vi "CmdExe.Launch Executable with Timeout, Abort, and Error Checks_V3.vi"(4 "StdIn":string, 5 "Cmd IN Ref":refnum<vi>, 6 "Setup":T1={"Timeout (s)"=60.0, "Show Cmd Win"=FALSE, "Error Check"={"StdOut_Ck"=FALSE, "StdOutErrMsgs"=["Error", "Unable to find device "], "StdErr_Ck"=FALSE, "RtnCode_Ck"=FALSE, "RtnCodePASS"=0}, "Log_En"=FALSE, "LogFileName"="", "LogDir"=path ""}, 7 "Output Ref":refnum<vi>, 8 "error in (no error)":errorcluster, 9 "Ignore StdErr":bool, 10 "Args":string, 11 "Executable":path=path "C:/MTE/FW Load and Display Cal/Config/Bin/utahev_0_7/lighthouse_configtool.exe") -> (0 "error out":errorcluster, 1 "Duration(s)":dbl, 2 "return code":i32, 3 "Data Out":string)   [LabVIEW 2024]
uses:
  CmdExe.Setup Params.ctl
  CmdExe.Output Error Check Setup.ctl
  Errors/Error.Error Code List.ctl
  Errors.lvlib
  <vilib>/KATE/Time/Time Utils.lvlib
  <vilib>/KATE/Files/File Utils.lvlib
panel:
  out "Cmd":string
  out "Done":bool
  # "Launch Exe"
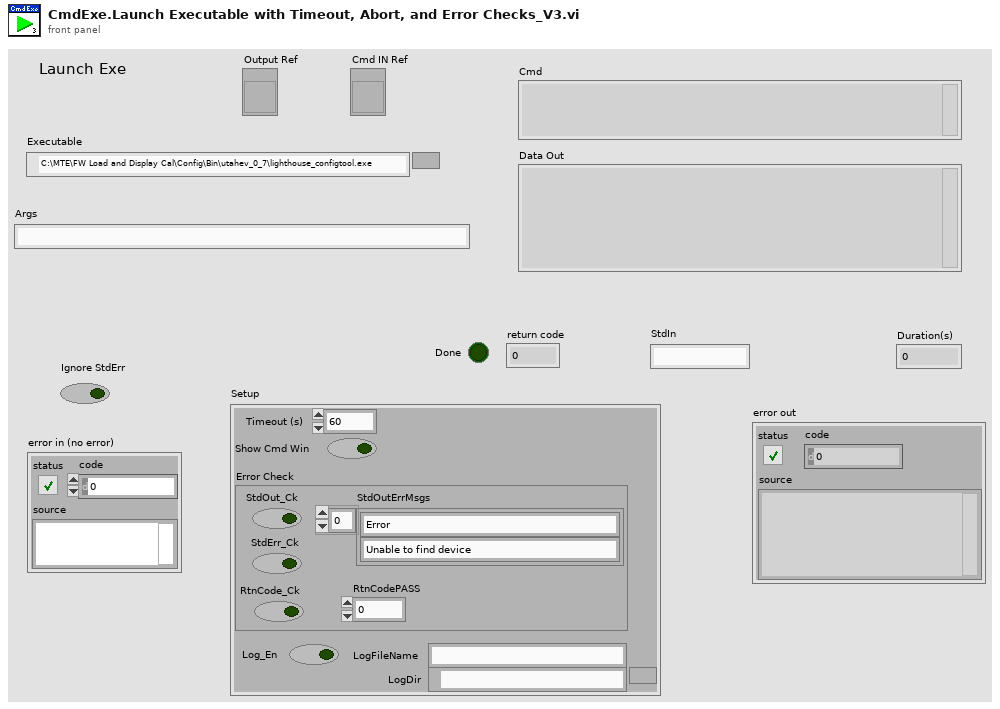
[diagram p1: front panel]
types:
  T1 = typedef "CmdExe.Setup Params.ctl" = cluster{"Timeout (s)":dbl, "Show Cmd Win":bool, "Error Check":T2, "Log_En":bool, "LogFileName":string, "LogDir":path}
  T2 = typedef "CmdExe.Output Error Check Setup.ctl" = cluster{"StdOut_Ck":bool, "StdOutErrMsgs":string[], "StdErr_Ck":bool, "RtnCode_Ck":bool, "RtnCodePASS":i32}
  T3 = enum16{"open", "replace", "create", "open or create", "replace or create", "replace or create with confirmation"}
  T4 = cluster{"Exe":string, "StdOut":string, "StdError":string, "LogFile":path, "Args":string, "TimedOut":bool, "RtnCode":i32, "LogEn":bool}
  T5 = typedef "EQMF.lvlib/Errors.lvlib/Error.Error Code List.ctl" = i32
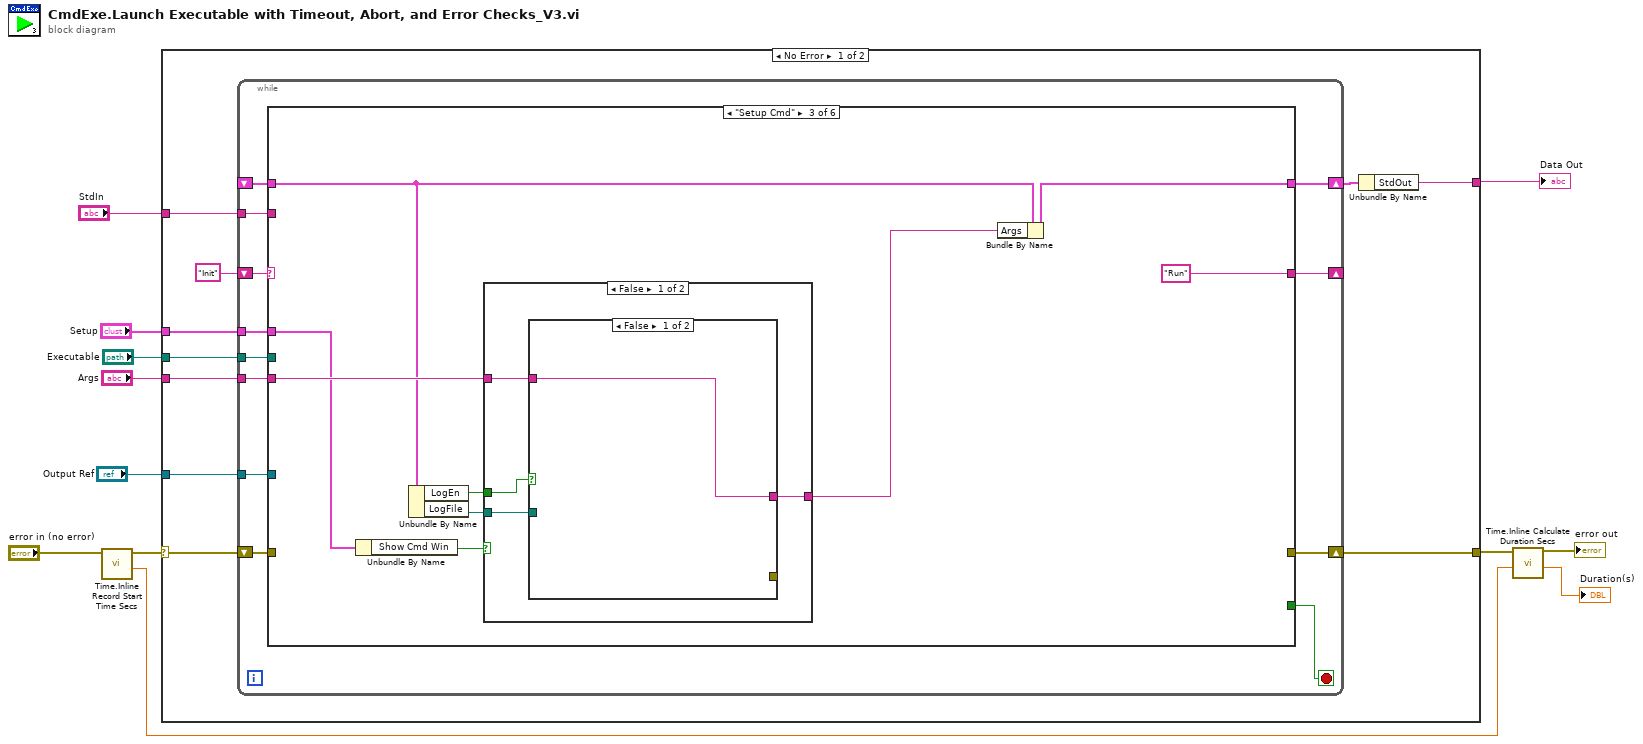
[diagram p0: block diagram]
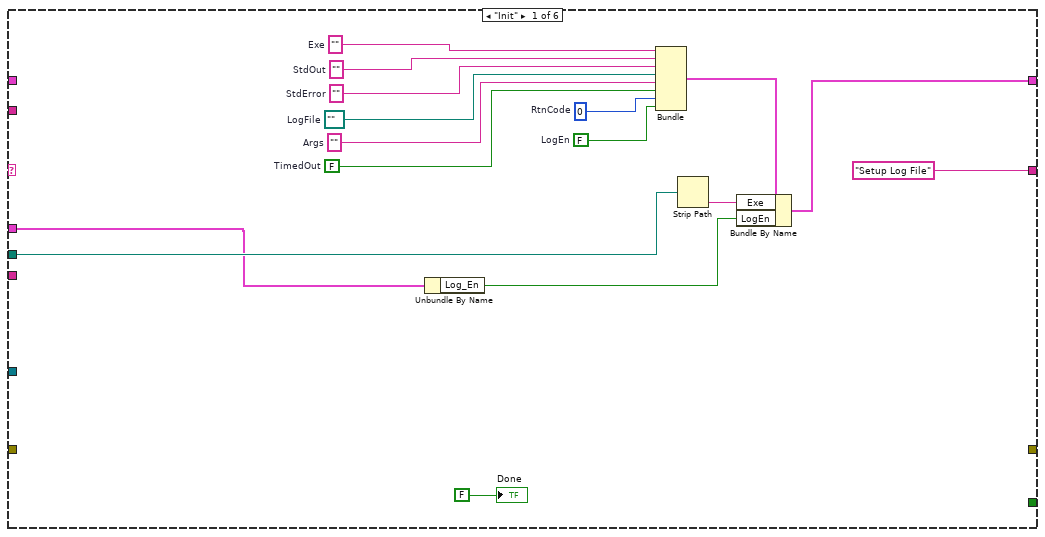
[diagram p2: hidden frame]
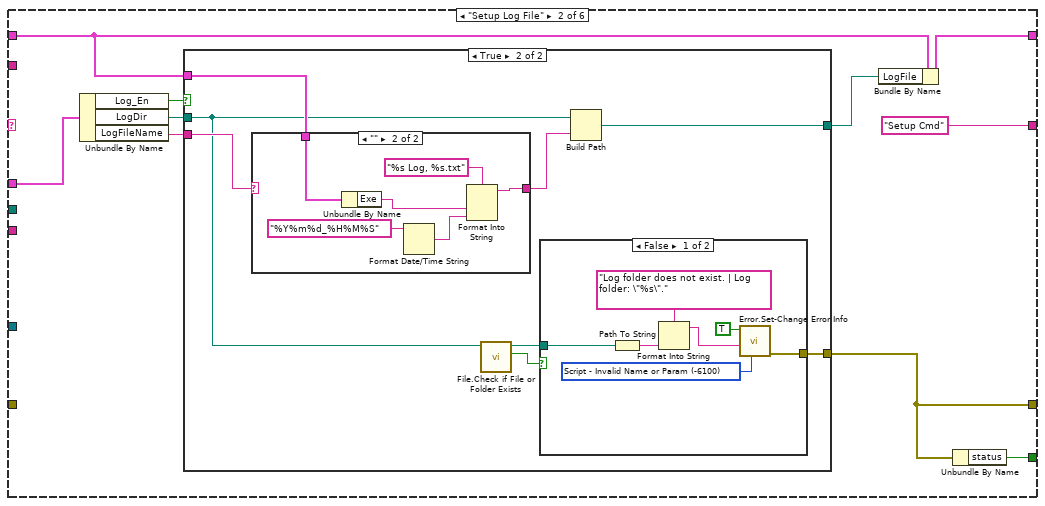
[diagram p3: hidden frame]
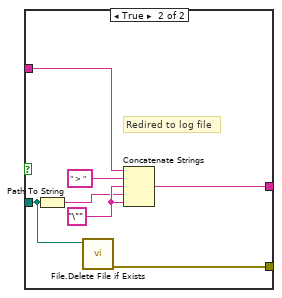
[diagram p7: hidden frame]
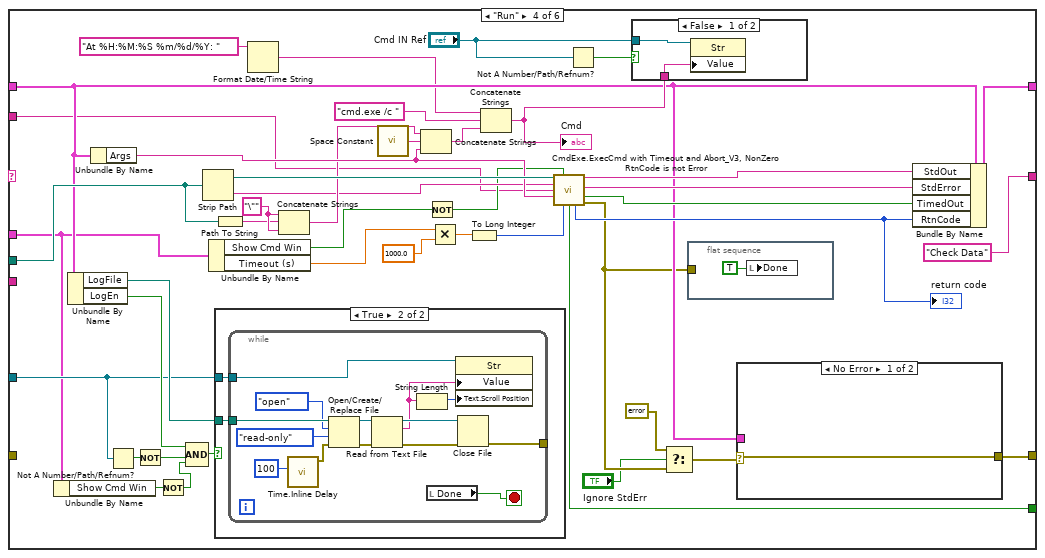
[diagram p9: hidden frame]
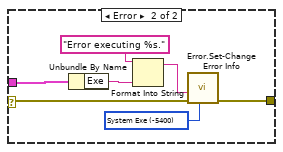
[diagram p10: hidden frame]
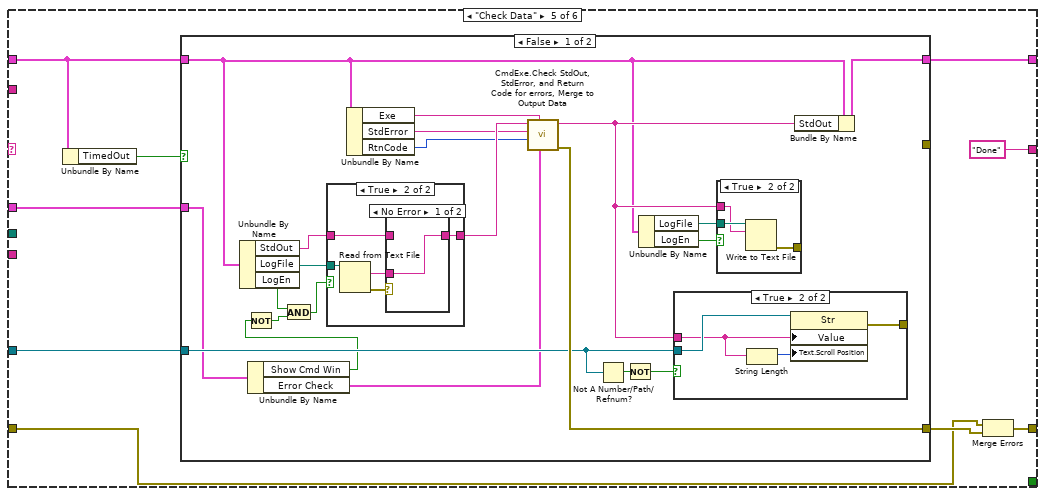
[diagram p13: hidden frame]
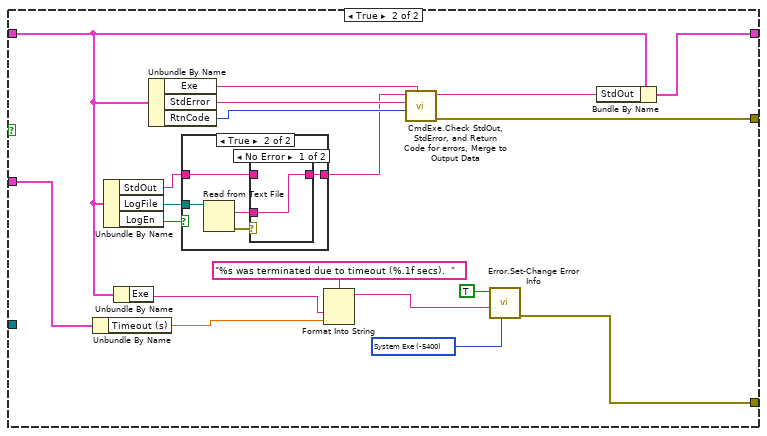
[diagram p18: hidden frame]
diagram:
  n1 = call <vilib>:"Time.Inline Record Start Time Secs.vi"("Error In Upper"="error in (no error)") -> ("Start(s)"=w9:dbl, "Error Out Upper"=w12:errorcluster)  [unwired: 8 in, 1 out]
  n2 = case shown="No Error" w12 {
    selector: w12 -> [w21 w252]
    tunnel: [w20 w252] -> w11
    tunnel: [w18 _] -> w10
    tunnel: "Executable" -> [w17 _]
    tunnel: "Args" -> [w16 _]
    tunnel: "Setup" -> [w15 _]
    tunnel: "Output Ref" -> [w14 _]
    tunnel: "StdIn" -> [w13 _]
    frame No Error {
      n3 = while {
        shift-right: [w32] -> w19
        shift-left: _ -> [w31]
        shift-right: [w24] -> _
        shift-left: "Init" -> [w34]
        shift-right: [w30] -> w20
        shift-left: w21 -> [w33]
        tunnel: w17 -> [w28]
        tunnel: w16 -> [w27]
        tunnel: w15 -> [w26]
        tunnel: w14 -> [w25]
        tunnel: w13 -> [w23]
        stop <- w29 stop-if-true
        n4 = case shown="\"Setup Cmd\"" w34 {
          tunnel: ["Setup Log File" "Setup Cmd" "Run" "Check Data" "Done" "Done"] -> w24
          tunnel: w33 -> [_ _ _ _ w176 w248]
          tunnel: [w39 w59 w90 w148 w184 w249] -> w32
          tunnel: [_ w52 _ w116 w178 w248] -> w30
          tunnel: w31 -> [_ w57 w85 w115 w182 w249]
          tunnel: [_ w51 _ w144 _ TRUE] -> w29
          tunnel: w28 -> [w42 _ _ w129 _ _]
          tunnel: w27 -> [_ _ w88 _ _ _]
          tunnel: w26 -> [w36 w56 w84 w110 w180 _]
          tunnel: w25 -> [_ _ _ w117 w183 _]
          tunnel: w23 -> [_ _ _ w107 _ _]
          frame "Init" {
            w37 = FALSE  # LogEn
            w38 = 0  # RtnCode
            w43 = FALSE  # TimedOut
            w44 = ""  # Args
            w45 = path ""  # LogFile
            w46 = ""  # StdError
            w47 = ""  # StdOut
            w49 = ""  # Exe
            n5 = Unbundle By Name(w36) -> ("Log_En"=w35:bool)
            n6 = Bundle("Exe"=w49, "StdOut"=w47, "StdError"=w46, "LogFile"=w45, "Args"=w44, "TimedOut"=w43, "RtnCode"=w38, "LogEn"=w37) -> (w40:T4)  [unwired: 1 in]
            n7 = Strip Path(path=w42) -> (name=w41:string)  [unwired: 1 out]
            n8 = Bundle By Name(cluster=w40, "Exe"=w41, "LogEn"=w35) -> (w39:T4)
            "Done" <- FALSE ("Done")
          }
          frame "Setup Log File" {
            n9 = Unbundle By Name(w56) -> ("Log_En"=w55:bool, "LogDir"=w54:path, "LogFileName"=w53:string)
            n10 = case shown="True" w55 {
              tunnel: [_ w68] -> w58
              tunnel: w57 -> [_ w66]
              tunnel: w54 -> [_ w62]
              tunnel: w53 -> [_ w65]
              tunnel: [_ w61] -> w52
              frame False {
              }
              frame True {
                n11 = case shown="\"\"" w65 {
                  selector: w65 -> [w76 _]
                  tunnel: [w76 w79] -> w67
                  tunnel: w66 -> [_ w78]
                  frame Default {
                  }
                  frame "" {
                    n12 = Unbundle By Name(w78) -> ("Exe"=w77:string)
                    n13 = Format Date/Time String(time format string (%c)="%Y%m%d_%H%M%S") -> (date/time string=w82:string)  [unwired: 2 in]
                    n14 = Format Into String(format string="%s Log, %s.txt", w77, w82) -> (resulting string=w79:string)  [unwired: 2 in, 1 out]
                  }
                }
                n15 = call <vilib>:"File.Check if File or Folder Exists.vi"("Path"=w62) -> ("Exists"=w63:bool, "Dup Path"=w64:path)  [unwired: 6 in, 3 out]
                n16 = case shown="False" w63 {
                  tunnel: [w69 _] -> w61
                  tunnel: w64 -> [w73 _]
                  frame False {
                    w71 = T5 -6100 items=["No Error"=0, "Abort"=-2, "Misc"=-5000, "Fixture Error"=-5100, "File IO - General"=-5200, "FIle IO - Config Error"=-5201, "Instrument - General"=-5300, "Instrument - Serial Com"=-5301, "Instrument - Camera"=-5302, "Instrument - PS"=-5303, "Instrument - Oscilloscope"=-5304, "Instrument - Function Gen"=-5305, "Instrument - Load"=-5306, "Instrument - Meter"=-5307, "Instrument - Power Control"=-5308, "Instrument - Motion"=-5309, "Instrument - RF"=-5310, "System Exe"=-5400, "Image Processing"=-5500, "Communication"=-5600, "Script - Syntax Error"=-6000, "Script - Invalid Name or Param"=-6100, "Script - Timeout"=-6200, "Invalid Data"=-6300] ("Std Code")
                    n17 = Path To String(path=w73) -> (string=w74:string)
                    n18 = Format Into String(format string="Log folder does not exist. | Log folder: \"%s\".", w74) -> (resulting string=w70:string)  [unwired: 2 in, 1 out]
                    n19 = call "Error.Set-Change Error Info.vi"("Std Code"=w71, "Description"=w70, "Set Error"=TRUE) -> ("error out"=w69:errorcluster)  [unwired: 8 in]
                  }
                  frame True {
                    # "Folders exist.\nNo error."
                  }
                }
                n20 = Build Path(base path=w62, name or relative path=w67) -> (appended path=w68:path)
              }
            }
            n21 = Bundle By Name(cluster=w57, "LogFile"=w58) -> (w59:T4)
            n22 = Unbundle By Name(w52) -> ("status"=w51:bool)
          }
          frame "Setup Cmd" {
            n23 = Unbundle By Name(w84) -> ("Show Cmd Win"=w83:bool)
            n24 = Unbundle By Name(w85) -> ("LogEn"=w86:bool, "LogFile"=w89:path)
            n25 = case shown="False" w83 {
              tunnel: w89 -> [w95 _]
              tunnel: w88 -> [w94 w104]
              tunnel: [w93 w104] -> w87
              tunnel: w86 -> [w92 _]
              frame False {
                n26 = case shown="False" w92 {
                  tunnel: w95 -> [_ w98]
                  tunnel: w94 -> [w96 w100]
                  tunnel: [w96 w99] -> w93
                  tunnel: [_ w97] -> _
                  frame False {
                  }
                  frame True {
                    w103 = "\""
                    # "Redired to log file"
                    n27 = Path To String(path=w98) -> (string=w102:string)
                    n28 = call "File.Delete File if Exists.vi"("Path"=w98) -> ("error out"=w97:errorcluster)  [unwired: 9 in, 1 out]
                    n29 = Concatenate Strings(w100, " > ", w103, w102, w103) -> (w99:string)
                  }
                }
              }
              frame True {
              }
            }
            n30 = Bundle By Name(cluster=w85, "Args"=w87) -> (w90:T4)
          }
          frame "Run" {
            w130 = "\""
            n31 = Unbundle By Name(w110) -> ("Show Cmd Win"=w109:bool)
            n32 = Unbundle By Name(w115) -> ("LogFile"=w138:path, "LogEn"=w122:bool)
            n33 = Unbundle By Name(w115) -> ("Args"=w131:string)
            n34 = Not A Number/Path/Refnum?(number/path/refnum=w117) -> (NaN/Path/Refnum?=w125:bool)
            n35 = Not(x=w125) -> (.not. x?=w124:bool)
            n36 = Not(x=w109) -> (.not. x?=w108:bool)
            n37 = Compound Arithmetic op=AND(w122, w124, w108) -> (w123:bool)
            n38 = Strip Path(path=w129) -> (stripped path=w137:path, name=w126:string)
            n39 = Unbundle By Name(w110) -> ("Show Cmd Win"=w120:bool, "Timeout (s)"=w121:dbl)
            n40 = Path To String(path=w129) -> (string=w128:string)
            n41 = case shown="True" w123 {
              tunnel: w138 -> [_ w160]
              tunnel: w117 -> [_ w161]
              frame False {
              }
              frame True {
                n42 = while {
                  tunnel: w161 -> [w167]
                  tunnel: w160 -> [w171]
                  tunnel: [w170] -> _
                  stop <- w166 stop-if-true
                  n43 = call <vilib>:"Time.Inline Delay.vi"("Wait(ms)"=u32 100) -> ("error out top"=w164:errorcluster)  [unwired: 9 in, 1 out]
                  n44 = Open/Create/Replace File(file path (use dialog)=w171, error in=w164, operation (0:open)=T3."open", access (0:read/write)=enum16{"read/write", "read-only", "write-only"}."read-only") -> (refnum out=w172:refnum<file>, error out=w175:errorcluster)  [unwired: 2 in, 1 out]
                  n45 = Read from Text File(file (use dialog)=w172, error in=w175) -> (refnum out=w173:refnum<file>, text=w163:string, error out=w174:errorcluster)  [unwired: 2 in, 1 out]
                  n46 = String Length(string=w163) -> (length=w162:i32)
                  n47 = local read "Done"() -> (w166:bool)
                  n48 = property class="Str"(reference=w167, "Value"=w163, "Text.Scroll Position"=w162) -> ()  [unwired: 1 in, 2 out]
                  n49 = Close File(refnum=w173, error in=w174) -> (error out=w170:errorcluster)  [unwired: 1 out]
                }
              }
            }
            n50 = Format Date/Time String(time format string (%c)="At %H:%M:%S %m/%d/%Y: ") -> (date/time string=w105:string)  [unwired: 2 in]
            n51 = Concatenate Strings(w130, w128, w130) -> (w127:string)
            n52 = call <vilib>:"Space Constant.vi"() -> ("String"=w134:string)
            n53 = Concatenate Strings(w127, w134, w131) -> (w135:string)
            n54 = Not(x=w120) -> (.not. x?=w119:bool)
            n55 = Multiply(x=w121, y=1000.0) -> (x*y=w143:dbl)
            n56 = To Long Integer(number=w143) -> (32bit integer=w141:i32)
            n57 = Concatenate Strings(w105, "cmd.exe /c ", w135) -> (w133:string)
            "Cmd" <- w133
            n58 = call "CmdExe.ExecCmd with Timeout and Abort_V3, NonZero RtnCode is not Error.vi"("Working Dir"=w137, "Run minimized? (T)"=w119, "Executable"=w126, "StdIn"=w107, "Arguements"=w131, "Timeout ms(-1)"=w141) -> ("STD OUT"=w118:string, "STD ERR"=w147:string, "Timed Out"=w146:bool, "Aborted"=w144:bool, "return code"=w132:i32, "error out"=w114:errorcluster)  [unwired: 4 in]
            "return code" <- w132
            n59 = Not A Number/Path/Refnum?(number/path/refnum="Cmd IN Ref") -> (NaN/Path/Refnum?=w140:bool)
            n60 = case shown="False" w140 {
              tunnel: "Cmd IN Ref" -> [w159 _]
              tunnel: w133 -> [w158 _]
              frame False {
                n61 = property class="Str"(reference=w159, "Value"=w158) -> ()  [unwired: 1 in, 2 out]
              }
              frame True {
              }
            }
            n62 = Select(t=errorcluster {"status"=FALSE, "code"=0, "source"=""}, s="Ignore StdErr", f=w114) -> (s? t:f=w113:errorcluster)
            n63 = flat-sequence {
              tunnel: w114 -> [_]
              frame #0 {
                n64 = local write "Done"(TRUE ("Done")) -> ()
              }
            }
            n65 = case shown="No Error" w113 {
              selector: w113 -> [w149 w152]
              tunnel: [w149 w151] -> w116
              tunnel: w115 -> [_ w150]
              frame No Error {
              }
              frame Error {
                w154 = T5 -5400 items=["No Error"=0, "Abort"=-2, "Misc"=-5000, "Fixture Error"=-5100, "File IO - General"=-5200, "FIle IO - Config Error"=-5201, "Instrument - General"=-5300, "Instrument - Serial Com"=-5301, "Instrument - Camera"=-5302, "Instrument - PS"=-5303, "Instrument - Oscilloscope"=-5304, "Instrument - Function Gen"=-5305, "Instrument - Load"=-5306, "Instrument - Meter"=-5307, "Instrument - Power Control"=-5308, "Instrument - Motion"=-5309, "Instrument - RF"=-5310, "System Exe"=-5400, "Image Processing"=-5500, "Communication"=-5600, "Script - Syntax Error"=-6000, "Script - Invalid Name or Param"=-6100, "Script - Timeout"=-6200, "Invalid Data"=-6300] ("Std Code")
                n66 = Unbundle By Name(w150) -> ("Exe"=w155:string)
                n67 = Format Into String(format string="Error executing %s.", w155) -> (resulting string=w153:string)  [unwired: 2 in, 1 out]
                n68 = call "Error.Set-Change Error Info.vi"("Std Code"=w154, "error in"=w152, "Description"=w153) -> ("error out"=w151:errorcluster)  [unwired: 8 in]
              }
            }
            n69 = Bundle By Name(cluster=w115, "StdOut"=w118, "StdError"=w147, "TimedOut"=w146, "RtnCode"=w132) -> (w148:T4)
          }
          frame "Check Data" {
            n70 = Unbundle By Name(w182) -> ("TimedOut"=w181:bool)
            n71 = case shown="False" w181 {
              tunnel: [w205 w227] -> w184
              tunnel: w182 -> [w189 w221]
              tunnel: [w200 w232] -> w177
              tunnel: w183 -> [w197 _]
              tunnel: w180 -> [w194 w237]
              tunnel: [_ w222] -> _
              frame False {
                n72 = Unbundle By Name(w189) -> ("StdOut"=w195:string, "LogFile"=w204:path, "LogEn"=w188:bool)
                n73 = Unbundle By Name(w194) -> ("Show Cmd Win"=w186:bool, "Error Check"=w193:T2)
                n74 = Not(x=w186) -> (.not. x?=w187:bool)
                n75 = And(x=w188, y=w187) -> (x .and. y?=w185:bool)
                n76 = case shown="True" w185 {
                  tunnel: w204 -> [_ w218]
                  tunnel: [w213 w216] -> w203
                  tunnel: w195 -> [w213 w214]
                  frame False {
                    (unwired) TRUE
                  }
                  frame True {
                    n77 = Read from Text File(file (use dialog)=w218) -> (text=w215:string, error out=w217:errorcluster)  [unwired: 3 in, 2 out]
                    n78 = case shown="No Error" w217 {
                      tunnel: [w219 w220] -> w216
                      tunnel: w215 -> [w219 _]
                      tunnel: w214 -> [_ w220]
                      frame No Error {
                      }
                      frame Error {
                      }
                    }
                  }
                }
                n79 = Unbundle By Name(w189) -> ("Exe"=w196:string, "StdError"=w202:string, "RtnCode"=w201:i32)
                n80 = call "CmdExe.Check StdOut, StdError, and Return Code for errors, Merge to Output Data.vi"("Error Check"=w193, "App Name"=w196, "Return Code"=w201, "StdError"=w202, "StdOut"=w203) -> ("error out"=w200:errorcluster, "Output Data"=w190:string)  [unwired: 5 in]
                n81 = Not A Number/Path/Refnum?(number/path/refnum=w197) -> (NaN/Path/Refnum?=w199:bool)
                n82 = Not(x=w199) -> (.not. x?=w198:bool)
                n83 = Unbundle By Name(w189) -> ("LogFile"=w192:path, "LogEn"=w191:bool)
                n84 = case shown="True" w198 {
                  tunnel: w197 -> [_ w211]
                  tunnel: w190 -> [_ w210]
                  tunnel: [_ w209] -> _
                  frame False {
                  }
                  frame True {
                    n85 = String Length(string=w210) -> (length=w212:i32)
                    n86 = property class="Str"(reference=w211, "Value"=w210, "Text.Scroll Position"=w212) -> (error out=w209:errorcluster)  [unwired: 1 in, 1 out]
                  }
                }
                n87 = case shown="True" w191 {
                  tunnel: w192 -> [_ w208]
                  tunnel: [_ w207] -> _
                  tunnel: w190 -> [_ w206]
                  frame False {
                    (unwired) TRUE
                  }
                  frame True {
                    n88 = Write to Text File(file (use dialog)=w208, text=w206) -> (error out=w207:errorcluster)  [unwired: 2 in, 2 out]
                  }
                }
                n89 = Bundle By Name(cluster=w189, "StdOut"=w190) -> (w205:T4)
              }
              frame True {
                w235 = T5 -5400 items=["No Error"=0, "Abort"=-2, "Misc"=-5000, "Fixture Error"=-5100, "File IO - General"=-5200, "FIle IO - Config Error"=-5201, "Instrument - General"=-5300, "Instrument - Serial Com"=-5301, "Instrument - Camera"=-5302, "Instrument - PS"=-5303, "Instrument - Oscilloscope"=-5304, "Instrument - Function Gen"=-5305, "Instrument - Load"=-5306, "Instrument - Meter"=-5307, "Instrument - Power Control"=-5308, "Instrument - Motion"=-5309, "Instrument - RF"=-5310, "System Exe"=-5400, "Image Processing"=-5500, "Communication"=-5600, "Script - Syntax Error"=-6000, "Script - Invalid Name or Param"=-6100, "Script - Timeout"=-6200, "Invalid Data"=-6300] ("Std Code")
                n90 = Unbundle By Name(w237) -> ("Timeout (s)"=w236:dbl)
                n91 = Unbundle By Name(w221) -> ("StdOut"=w224:string, "LogFile"=w226:path, "LogEn"=w225:bool)
                n92 = Unbundle By Name(w221) -> ("Exe"=w238:string)
                n93 = Unbundle By Name(w221) -> ("Exe"=w229:string, "StdError"=w231:string, "RtnCode"=w230:i32)
                n94 = case shown="True" w225 {
                  tunnel: w226 -> [_ w245]
                  tunnel: [w240 w243] -> w223
                  tunnel: w224 -> [w240 w241]
                  frame False {
                    (unwired) TRUE
                  }
                  frame True {
                    n95 = Read from Text File(file (use dialog)=w245) -> (text=w242:string, error out=w244:errorcluster)  [unwired: 3 in, 2 out]
                    n96 = case shown="No Error" w244 {
                      tunnel: [w246 w247] -> w243
                      tunnel: w242 -> [w246 _]
                      tunnel: w241 -> [_ w247]
                      frame No Error {
                      }
                      frame Error {
                      }
                    }
                  }
                }
                n97 = Format Into String(format string="%s was terminated due to timeout (%.1f secs).  ", w238, w236) -> (resulting string=w233:string)  [unwired: 2 in, 1 out]
                n98 = call "CmdExe.Check StdOut, StdError, and Return Code for errors, Merge to Output Data.vi"("App Name"=w229, "Return Code"=w230, "StdError"=w231, "StdOut"=w223) -> ("error out"=w222:errorcluster, "Output Data"=w228:string)  [unwired: 6 in]
                n99 = call "Error.Set-Change Error Info.vi"("Std Code"=w235, "Description"=w233, "Set Error"=TRUE) -> ("error out"=w232:errorcluster)  [unwired: 8 in]
                n100 = Bundle By Name(cluster=w221, "StdOut"=w228) -> (w227:T4)
              }
            }
            n101 = Merge Errors(w176, w177) -> (w178:errorcluster)
          }
          frame "Done", Default {
          }
        }
      }
      n102 = Unbundle By Name(w19) -> ("StdOut"=w18:string)
    }
    frame Error {
    }
  }
  "Data Out" <- w10
  n103 = call <vilib>:"Time.Inline Calculate Duration Secs.vi"("Start(Sec)"=w9, "Error In Top"=w11) -> ("Duration(s)"=→"Duration(s)":dbl, "Error Out Top"=→"error out":errorcluster)  [unwired: 7 in, 1 out]
